vi "Get Children ALL.vi"(8 "error in":errorcluster, 10 "Parent Tag":string, 11 "Tree Reference":refnum<vi>) -> (0 "error out":errorcluster, 2 "Children Tags":string[](array[string]), 3 "Tree Reference":refnum<vi>)   [LabVIEW 2014, in "DSLV_Tree.lvlib"]
uses:
  DSLV_Tree.lvlib
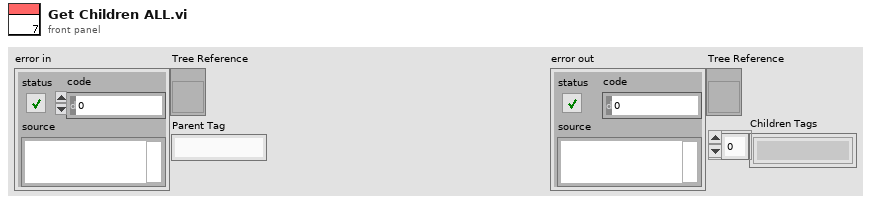
[diagram p1: front panel]
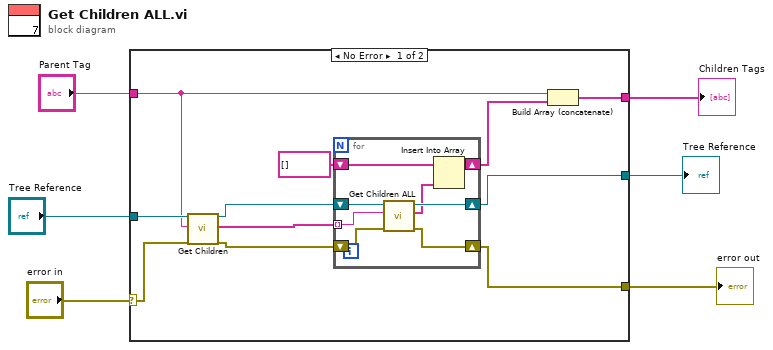
[diagram p0: block diagram]
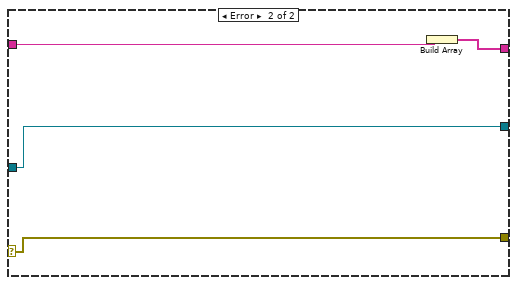
[diagram p2: hidden frame]
diagram:
  n1 = case shown="No Error" "error in" {
    selector: "error in" -> [w7 w26]
    tunnel: [w17 w26] -> w6
    tunnel: [w16 w27] -> w5
    tunnel: "Tree Reference" -> [w15 w27]
    tunnel: "Parent Tag" -> [w14 w29]
    tunnel: [w12 w28] -> w2
    frame No Error {
      n2 = call "Get Children.vi"("Tree Reference In"=w15, "Parent Tag"=w14, "error in (no error)"=w7) -> ("Tree Reference Out"=w11:refnum<vi>, "Children Tags"=w10:string[], "error out"=w8:errorcluster)  [unwired: 14 in]
      n3 = for {
        shift-right: [w25] -> w16
        shift-left: w11 -> [w24]
        shift-right: [w23] -> w17
        shift-left: w8 -> [w22]
        tunnel: w10 -> [w21] mode=indexing
        shift-right: [w19] -> w13
        shift-left: string[] [] -> [w18]
        n4 = call "Get Children ALL.vi"("error in"=w22, "Parent Tag"=w21, "Tree Reference"=w24) -> ("error out"=w23:errorcluster, "Children Tags"=w20:string[], "Tree Reference"=w25:refnum<vi>)  [unwired: 6 in]
        n5 = Insert Into Array(array=w18, new element=w20) -> (w19:string[])  [unwired: 1 in]
      }
      n6 = Build Array (concatenate)(w14, w13) -> (w12:string[])
    }
    frame Error {
      n7 = Build Array(w29) -> (w28:string[])
    }
  }
  "error out" <- w6
  "Tree Reference" <- w5
  "Children Tags" <- w2
